vi "Get DSF File Version.vi"() -> (3 "dsf":T1)   [LabVIEW 2021, in "DSF Core.lvlib" / "Configuration Session.lvclass"]
uses:
  Configuration Session.lvclass
  Typedefs/DSF Version Info.ctl
  DSF Core.lvlib
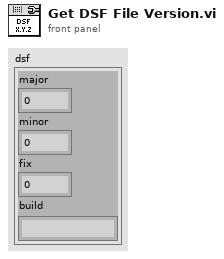
[diagram p1: front panel]
types:
  T1 = typedef "DSF Core.lvlib/DSF Version Info.ctl" = cluster{"major":u32, "minor":u32, "fix":u32, "build":string}
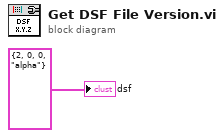
[diagram p0: block diagram]
diagram:
  "dsf" <- T1 {"major"=2, "minor"=0, "fix"=0, "build"="alpha"} ("dsf")
